vi "ini_save_variables.vi"(8 "error in":errorcluster, 10 "VI to store":refnum<vi>[](array[refnum]), 11 "objects":refnum<vi>[](array[refnum])) -> (0 "error out":errorcluster)   [LabVIEW 2020]
doc: "Call this to reload referenced objects from INI files."
uses:
  <vilib>/Utility/config.llb/NI_LVConfig.lvlib
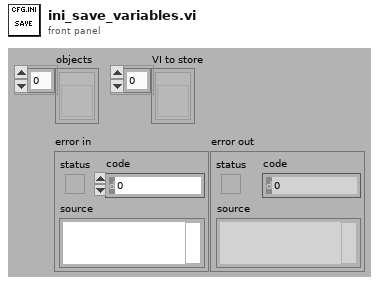
[diagram p1: front panel]
types:
  T1 = typedef "ini_parse_row.ctl" = cluster{"ini section":string, "ini key":string, "ini default":string, "control ref":refnum<vi>, "uid":i32, "vi ref":refnum<vi>}
  T2 = typedef "NI_LVConfig.lvlib/Config Data RefNum.ctl" = refnum<k1>
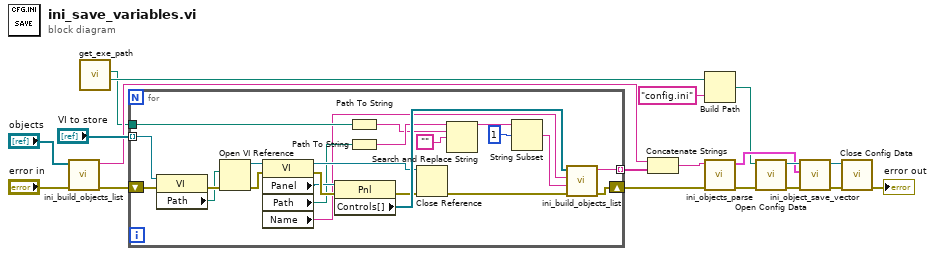
[diagram p0: block diagram]
diagram:
  n1 = call "ini_build_objects_list.vi"("error in"="error in", "objects"="objects") -> ("error out"=w10:errorcluster, "objects list"=w7:string)  [unwired: 8 in]
  n2 = call "get_exe_path.vi"() -> ("directory path"=w11:path, "application root path"=w6:path)  [unwired: 2 out]
  n3 = for {
    tunnel: "VI to store" -> [w36] mode=indexing
    shift-right: [w40] -> w1
    shift-left: w10 -> [w37]
    tunnel: [w38] -> w8 mode=indexing
    tunnel: w6 -> [w28]
    n4 = property class="VI"(reference=w36, error in=w37) -> (error out=w35:errorcluster, "Path"=w34:path)  [unwired: 1 out]
    n5 = Open VI Reference(vi path=w34, error in (no error)=w35) -> (vi reference=w32:refnum<vi>, error out=w33:errorcluster)  [unwired: 4 in]
    n6 = property class="VI"(reference=w32, error in=w33) -> (reference out=w29:refnum<vi>, error out=w42:errorcluster, "Panel"=w41:refnum<vi>, "Path"=w27:path, "Name"=w20:string)
    n7 = property class="Pnl"(reference=w41, error in=w42) -> (error out=w31:errorcluster, "Controls[]"=w39:refnum<vi>[])  [unwired: 1 out]
    n8 = Path To String(path=w28) -> (string=w25:string)
    n9 = Path To String(path=w27) -> (string=w26:string)
    n10 = Close Reference(reference=w29, error in (no error)=w31) -> (error out=w30:errorcluster)
    n11 = Search and Replace String(input string=w26, search string=w25, replace string="" ("replace string (\"\")")) -> (result string=w23:string)  [unwired: 5 in, 3 out]
    n12 = String Subset(string=w23, offset (0)=1) -> (substring=w21:string)  [unwired: 1 in]
    n13 = call "ini_build_objects_list.vi"("error in"=w30, "VI rel path (empty)"=w21, "VI name (empty)"=w20, "objects"=w39) -> ("error out"=w40:errorcluster, "objects list"=w38:string)  [unwired: 6 in]
  }
  n14 = Concatenate Strings(w7, w8) -> (w2:string)
  n15 = Build Path(base path=w11, name or relative path="config.ini") -> (appended path=w3:path)
  n16 = call "ini_objects_parse.vi"("error in"=w1, "items command"=w2) -> ("error out"=w14:errorcluster, "ini items"=w13:T1[])  [unwired: 8 in]
  n17 = call <vilib>:"Open Config Data.vi"("error in (no error)"=w14, "configuration file path"=w3) -> ("error out"=w15:errorcluster, "refnum"=w18:T2)  [unwired: 7 in, 1 out]
  n18 = call "ini_object_save_vector.vi"("error in"=w15, "objects to save"=w13, "refnum in"=w18) -> ("error out"=w17:errorcluster, "refnum out"=w16:T2)  [unwired: 7 in]
  n19 = call <vilib>:"Close Config Data.vi"("error in (no error)"=w17, "refnum"=w16) -> ("error out"=→"error out":errorcluster)  [unwired: 8 in, 1 out]
